vi "Process.vi"(8 "error in":errorcluster, 11 "Plugin in":refnum<class "PXIe-4113 DC Power Supply NI-DCPower Runtime Plugin PowerSupply.lvclass">) -> (0 "error out":errorcluster, 3 "Plugin out":refnum<class "PXIe-4113 DC Power Supply NI-DCPower Runtime Plugin PowerSupply.lvclass">)   [LabVIEW 2026, in "PXIe-4113 DC Power Supply NI-DCPower Runtime Plugin PowerSupply.lvlib" / "PXIe-4113 DC Power Supply NI-DCPower Runtime Plugin PowerSupply.lvclass"]
uses:
  PXIe-4113 DC Power Supply NI-DCPower Runtime Plugin PowerSupply.lvclass
  C:/Program Files/National Instruments/LabVIEW 2026/vi.lib/FlexLogger/SDK/PluginSDK.lvlibp/PEFClasses/SDK/Plugin/Plugin.lvclass
  PXIe-4113 DC Power Supply NI-DCPower Runtime Plugin PowerSupply.lvclass/PXIe-4113 DC Power Supply NI-DCPower Runtime Plugin PowerSupply.ctl
  <vilib>/FlexLogger/SDK/PluginSDK.lvlibp/PEFClasses/SDK/Plugin/DataHelpers/Write 1D DBL (NChan 1Sample).vi
  C:/Program Files/National Instruments/LabVIEW 2026/vi.lib/FlexLogger/SDK/PluginSDK.lvlibp/PEFClasses/SDK/Processing Element/Processing Element.lvclass
  C:/Users/krael/OneDrive - Emerson/Documents/LabVIEW Projects/FlexLogger IO Plug-ins/PXIe-4113 DC Power Supply NI-DCPower Runtime Plugin PowerSupply/PXIe-4113 DC Power Supply NI-DCPower Runtime Plugin PowerSupply.lvclass
  <vilib>/FlexLogger/SDK/PluginSDK.lvlibp/PEFClasses/SDK/Plugin/Plugin.lvclass
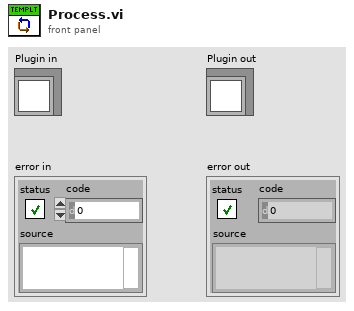
[diagram p1: front panel]
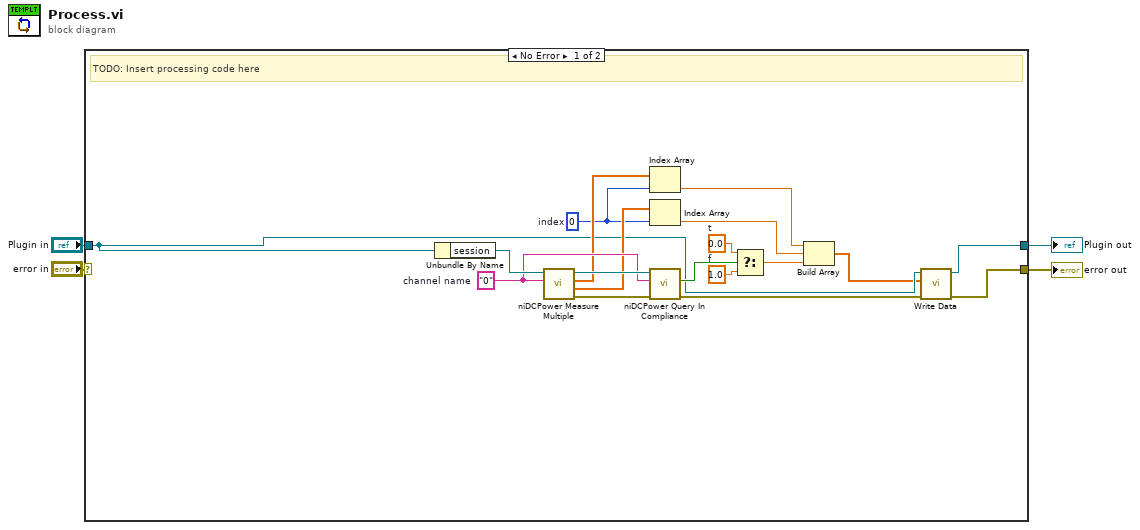
[diagram p0: block diagram]
diagram:
  n1 = case shown="No Error" "error in" {
    selector: "error in" -> [_ w23]
    tunnel: [w6 w24] -> w4
    tunnel: "Plugin in" -> [w9 w24]
    tunnel: [w5 w23] -> w1
    frame No Error {
      w13 = 1.0  # f
      w15 = 0.0  # t
      w16 = 0  # index
      w20 = "0"  # channel name
      # "TODO: Insert processing code here"
      n2 = Unbundle By Name(w9) -> ("session"=w22:refnum<k15>)
      n3 = call <instrlib>:"niDCPower Measure Multiple.vi"("channel name"=w20, "instrument handle"=w22) -> ("error out"=w19:errorcluster, "current measurements"=w17:dbl[], "voltage measurements"=w18:dbl[], "instrument handle out"=w21:refnum<k15>)  [unwired: 6 in]
      n4 = Index Array(array=w18, index=w16) -> (element=w12:dbl)
      n5 = Index Array(array=w17, index=w16) -> (element=w11:dbl)
      n6 = call <instrlib>:"niDCPower Query In Compliance.vi"("error in (no error)"=w19, "channel name"=w20, "instrument handle"=w21) -> ("error out"=w7:errorcluster, "in compliance?"=w14:bool)  [unwired: 6 in, 1 out]
      n7 = Select(t=w15, s=w14, f=w13) -> (s? t:f=w10:dbl)
      n8 = Build Array(w12, w11, w10) -> (w8:dbl[])
      n9 = call-poly <vilib>:"Write Data.vi"("error in (no error)"=w7, "Data"=w8, "Plugin in"=w9) -> ("error out"=w5:errorcluster, "Plugin out"=w6:refnum<class "PXIe-4113 DC Power Supply NI-DCPower Runtime Plugin PowerSupply.lvclass">)  [unwired: 7 in]
    }
    frame Error {
    }
  }
  "error out" <- w1
  "Plugin out" <- w4
